vi "tirf-lock-globals.vi"() -> ()   [LabVIEW 2014]
panel:
  in  "Channels for x,y, and power supply":tag
  in  "Sampling Rate (Hz)":dbl=100.0
  in  "Minimum Value":dbl=-10.0
  in  "Maximum Value":dbl=10.0 format="%_2f"
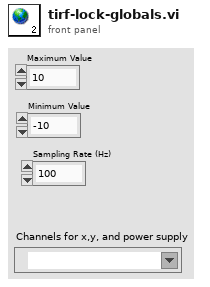
[diagram p1: front panel]
diagram:
